vi "q1 tf to state space.vi"() -> ()   [LabVIEW 2018]
uses:
  <vilib>/addons/Control Design/_Utility/Rendering.llb/Rendering Transfer Function Options.ctl
  <vilib>/addons/Control Design/_Model Construction/Model Creation.llb/Model Creation SubVI/cd_Create Transfer Function Model.vi
  <vilib>/addons/Control Design/_Utility/Model Viewer.llb/Model Viewer SubVI/cd_Draw Transfer Function Equation (TF).vi
  <vilib>/addons/Control Design/_Model Conversions/Model Type.llb/Model Conversion SubVI/cd_Convert Transfer Function to State-Space Model.vi
  <vilib>/addons/Control Design/_Utility/Model Viewer.llb/Model Viewer SubVI/cd_Draw State-Space Equation (SS).vi
  <vilib>/addons/Control Design/_Model Construction/NI_LinSys_Model Creation.lvlib
  <vilib>/addons/Control Design/_Utility/NI_CD_Model Viewer.lvlib
  <vilib>/addons/Control Design/_Model Conversions/NI_CD_Model Type.lvlib
  <vilib>/addons/Control Design/_Utility/NI_LinSys_Rendering.lvlib
panel:
  out "State Space":picture
  out "Transfer Function":picture
  in  "Display Format":T1 items=["Descending", "Ascending", "Negative Power"]
  in  "Denominator":dbl[](array[numeric]) format="%#.5g"
  in  "Numerator":dbl[](array[numeric]) format="%#.5g"
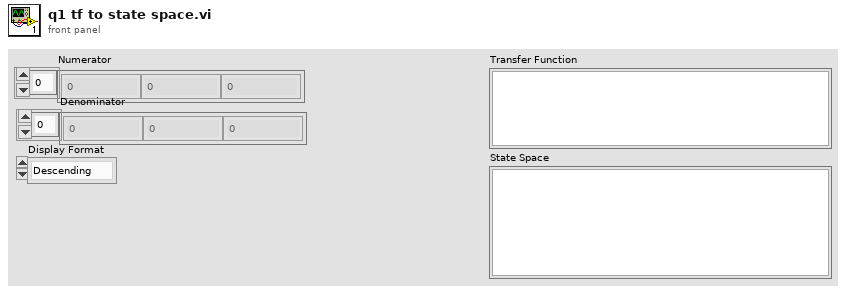
[diagram p1: front panel]
types:
  T1 = typedef "NI_LinSys_Rendering.lvlib/Rendering Transfer Function Options.ctl" = u16
  T2 = typedef "NI_LinSys_Model Typedefs.lvlib/CD Transfer Function Model (MIMO).ctl" = cluster{"properties":T3, "transfer function(s)":T4[][]}
  T3 = typedef "NI_LinSys_Model Typedefs.lvlib/CD General Elements.ctl" = cluster{"Model name":string, "Input names":string[], "Output names":string[], "Input Delays":dbl[], "Output Delays":dbl[], "Sampling Time":dbl, "Notes":string}
  T4 = typedef "NI_LinSys_Model Typedefs.lvlib/CD Transfer Function Model (SISO).ctl" = cluster{"Numerator":dbl[], "Denominator":dbl[], "delay":dbl}
  T5 = typedef "NI_LinSys_Model Typedefs.lvlib/CD State Space Model (MIMO).ctl" = cluster{"properties":T3, "A":dbl[][], "B":dbl[][], "C":dbl[][], "D":dbl[][], "StateNames":string[], "Transport Delay":dbl[][]}
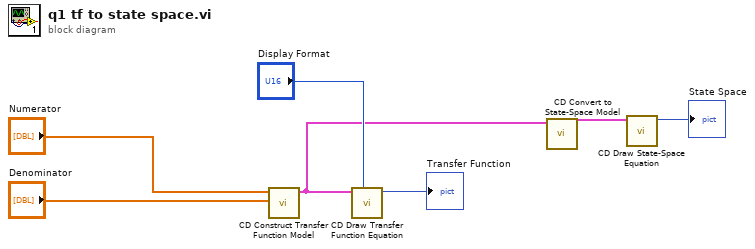
[diagram p0: block diagram]
diagram:
  n1 = call-poly <vilib>:"CD Construct Transfer Function Model.vi"("Denominator"="Denominator", "Numerator"="Numerator") -> ("Transfer Function Model"=w3:T2)  [unwired: 8 in, 1 out]
  n2 = call-poly <vilib>:"CD Draw Transfer Function Equation.vi"("Display Format"="Display Format", "Transfer Function Model"=w3) -> ("Equation"=→"Transfer Function":picture)  [unwired: 7 in, 2 out]
  n3 = call-poly <vilib>:"CD Convert to State-Space Model.vi"("Transfer Function Model"=w3) -> ("State-Space Model"=w2:T5)  [unwired: 9 in, 1 out]
  n4 = call-poly <vilib>:"CD Draw State-Space Equation.vi"("State-Space Model"=w2) -> ("Equation"=→"State Space":picture)  [unwired: 8 in, 2 out]
